vi "3KantVipOp_SubVI.vi"(0 "Shift 1 in":bool, 1 "Antal iterationer pr. stepper":i32, 5 "Loops shift in":i32, 7 "BUND!":bool, 9 "Index step array shift in":i32[](array[numeric]), 12 "Shift 2 in":bool, 13 "Shift 3 in":bool) -> (2 "Loops shift out":i32, 3 "Enable 1":bool, 4 "Index step array shift ud":i32[](array[numeric]), 6 "Shift 2 ud":bool, 8 "Enable 2":bool, 10 "Shift 3 ud":bool, 14 "Enable 3":bool, 15 "Direction":bool)   [LabVIEW 2019]
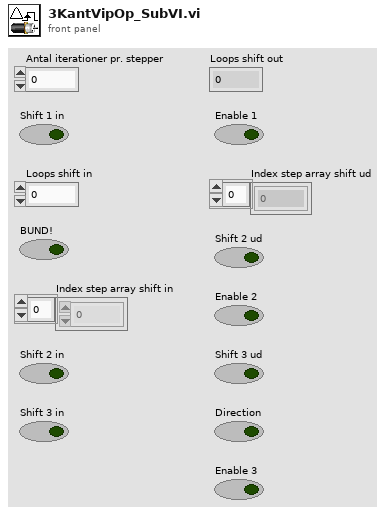
[diagram p1: front panel]
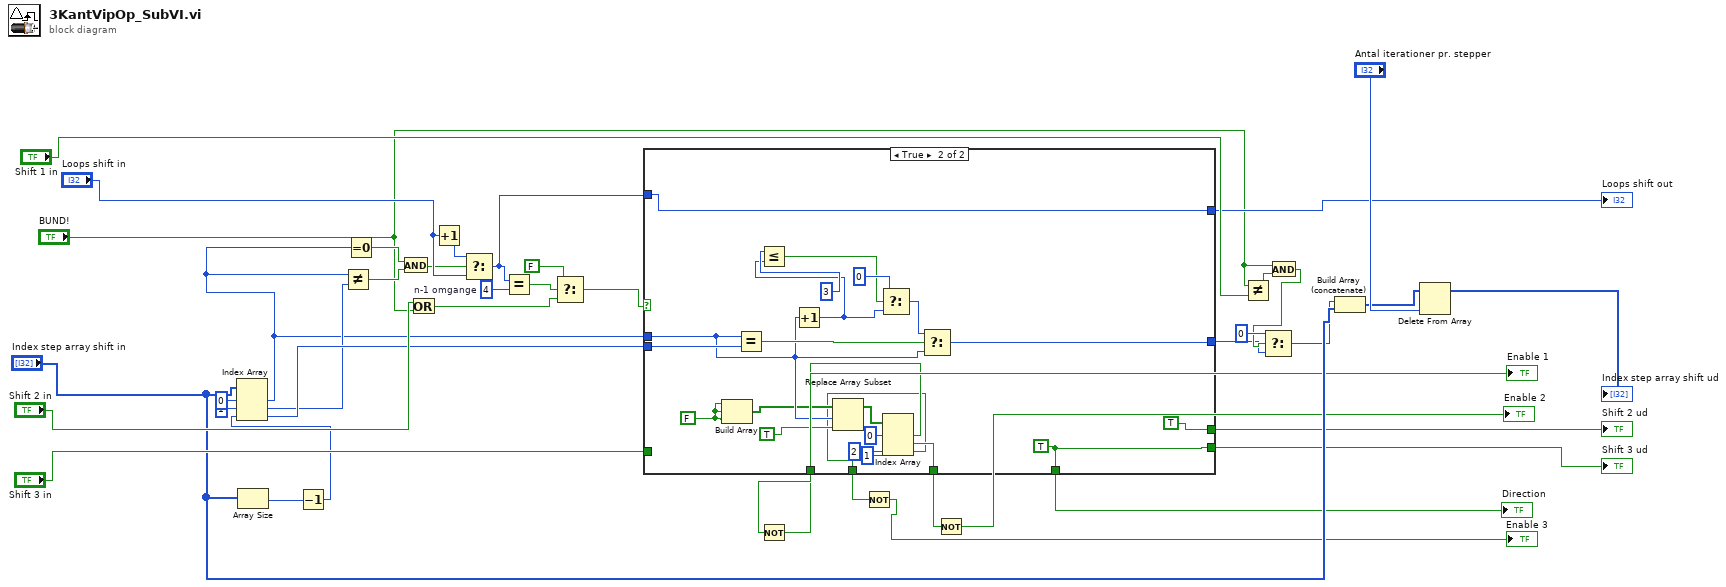
[diagram p0: block diagram]
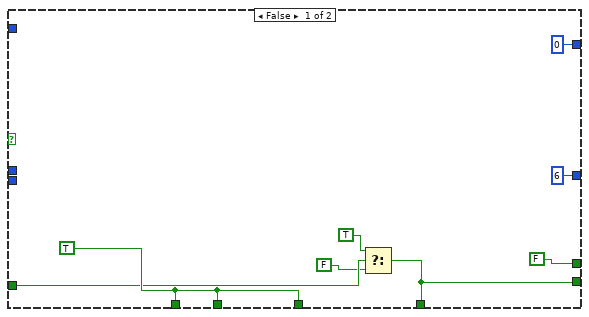
[diagram p2: hidden frame]
diagram:
  w13 = 4  # n-1 omgange
  n1 = Array Size(array="Index step array shift in") -> (size(s)=w33:i32)
  n2 = Decrement(x=w33) -> (x-1=w34:i32)
  n3 = Index Array(array="Index step array shift in", index #1=0 ("index"), index #2=1 ("index"), index #3=w34) -> (element #1=w30:i32, element #2=w32:i32, element #3=w35:i32)
  n4 = Not Equal?(x=w30, y=w32) -> (x != y?=w8:bool)
  n5 = Equal To 0?(x=w30) -> (x = 0?=w7:bool)
  n6 = And(x=w7, y=w8) -> (x .and. y?=w9:bool)
  n7 = Or(x="Shift 2 in", y="BUND!") -> (x .or. y?=w15:bool)
  n8 = Increment(x="Loops shift in") -> (x+1=w10:i32)
  n9 = Select(t=w10, s=w9, f="Loops shift in") -> (s? t:f=w12:i32)
  n10 = Equal?(x=w12, y=w13) -> (x = y?=w14:bool)
  n11 = Select(t=FALSE, s=w14, f=w15) -> (s? t:f=w16:bool)
  n12 = case shown="True" w16 {
    tunnel: w35 -> [_ w71]
    tunnel: w30 -> [_ w61]
    tunnel: [6 ("t") w67] -> w1
    tunnel: [FALSE TRUE ("BUND!")] -> w6
    tunnel: [0 w63] -> w11
    tunnel: w12 -> [_ w63]
    tunnel: [w46 w53] -> w21
    tunnel: [w46 w51] -> w22
    tunnel: [w46 w52] -> w25
    tunnel: [w42 w50] -> w18
    tunnel: "Shift 3 in" -> [w45 _]
    tunnel: [w42 w50] -> w19
    frame False {
      w46 = TRUE
      n13 = Select(t=TRUE, s=w45, f=FALSE) -> (s? t:f=w42:bool)
    }
    frame True {
      w50 = TRUE ("BUND!")
      w59 = FALSE
      n14 = Build Array(w59, w59, w59) -> (w60:bool[])
      n15 = Equal?(x=w61, y=w71) -> (x = y?=w70:bool)
      n16 = Increment(x=w61) -> (x+1=w64:i32)
      n17 = Less Or Equal?(x=3, y=w64) -> (x <= y?=w66:bool)
      n18 = Replace Array Subset(array=w60, new element=TRUE, index=w61) -> (w57:bool[])
      n19 = Select(t=0, s=w66, f=w64) -> (s? t:f=w69:i32)
      n20 = Index Array(array=w57, index #1=0 ("index"), index #2=1 ("index"), index #3=2 ("index")) -> (element #1=w53:bool, element #2=w52:bool, element #3=w51:bool)
      n21 = Select(t=w69, s=w70, f=w61) -> (s? t:f=w67:i32)
    }
  }
  "Shift 3 ud" <- w19
  "Direction" <- w18
  "Loops shift out" <- w11
  "Shift 2 ud" <- w6
  n22 = Not(x=w21) -> (.not. x?=→"Enable 1":bool)
  n23 = Not(x=w22) -> (.not. x?=→"Enable 3":bool)
  n24 = Not(x=w25) -> (.not. x?=→"Enable 2":bool)
  n25 = Not Equal?(x="BUND!", y="Shift 1 in") -> (x != y?=w2:bool)
  n26 = And(x="BUND!", y=w2) -> (x .and. y?=w3:bool)
  n27 = Select(t=0, s=w3, f=w1) -> (s? t:f=w26:i32)
  n28 = Build Array (concatenate)(w26, "Index step array shift in") -> (w27:i32[])
  n29 = Delete From Array(array=w27, index="Antal iterationer pr. stepper") -> (array with subset deleted=→"Index step array shift ud":i32[])  [unwired: 1 in, 1 out]
